vi "Settings cluster Broadcast.vi"(8 "error in (no error)":errorcluster, 10 "Settings cluster":T1={"Defaults"={"Default User"=0.0, "VISA Resource Name "="Tracker", "Histogram parameters"={"max"=300.0, "min"=0.0, "# bins"=10, "threshold"=8.0, "thr. type"=enum."higher accepted"}}, "Recording and saving"={"Researcher name"="Researcher", "Name prefix"="Track", "Data post-processing"={"Filter type"=enum."Savitzky-Golay", "Length"=31, "Order"=3}, "Stop at"=0.0, "\"Stop at\" enabled"=FALSE, "Default save folder path"=path "", "Acquisition FPS"=enum."Max"}, "Geometry"={"Sensor board size"=enum."Large", "Bridge swap"=FALSE, "Twisted neck"=FALSE, "Bridge H. offset"=30.0, "Bridge V. offset"=75.0, "Magnets orientation"=0.0, "Cage type"=0, "Cage parameters"={"Round"=variant, "Square"=variant, "Donut-maze"=variant, "T-maze"=variant, "Sociability-maze"=variant}}, "IO parameters"={"IO general config."=12, "IO 1 configuration"=1, "IO 2 configuration"=1, "IO 3 configuration"=0, "IO 4 configuration"=0, "Activate ext. RS-232"=0, "IO inversion config."=0, "Sync capability"=1}, "Conditions presets array"=[{"Enabled"=FALSE, "Name"="", "Specifier(s)"=[], "Response"={"Response type"=enum."Air puff", "TTL port"=enum."Port 1", "TTL pulse length, ms"=0.0}, "Has been set"=FALSE}, {"Enabled"=FALSE, "Name"="", "Specifier(s)"=[], "Response"={"Response type"=enum."Air puff", "TTL port"=enum."Port 1", "TTL pulse length, ms"=0.0}, "Has been set"=FALSE}, {"Enabled"=FALSE, "Name"="", "Specifier(s)"=[], "Response"={"Response type"=enum."Air puff", "TTL port"=enum."Port 1", "TTL pulse length, ms"=0.0}, "Has been set"=FALSE}, {"Enabled"=FALSE, "Name"="", "Specifier(s)"=[], "Response"={"Response type"=enum."Air puff", "TTL port"=enum."Port 1", "TTL pulse length, ms"=0.0}, "Has been set"=FALSE}, {"Enabled"=FALSE, "Name"="", "Specifier(s)"=[], "Response"={"Response type"=enum."Air puff", "TTL port"=enum."Port 1", "TTL pulse length, ms"=0.0}, "Has been set"=FALSE}, {"Enabled"=FALSE, "Name"="", "Specifier(s)"=[], "Response"={"Response type"=enum."Air puff", "TTL port"=enum."Port 1", "TTL pulse length, ms"=0.0}, "Has been set"=FALSE}, {"Enabled"=FALSE, "Name"="", "Specifier(s)"=[], "Response"={"Response type"=enum."Air puff", "TTL port"=enum."Port 1", "TTL pulse length, ms"=0.0}, "Has been set"=FALSE}, {"Enabled"=FALSE, "Name"="", "Specifier(s)"=[], "Response"={"Response type"=enum."Air puff", "TTL port"=enum."Port 1", "TTL pulse length, ms"=0.0}, "Has been set"=FALSE}, {"Enabled"=FALSE, "Name"="", "Specifier(s)"=[], "Response"={"Response type"=enum."Air puff", "TTL port"=enum."Port 1", "TTL pulse length, ms"=0.0}, "Has been set"=FALSE}, {"Enabled"=FALSE, "Name"="", "Specifier(s)"=[], "Response"={"Response type"=enum."Air puff", "TTL port"=enum."Port 1", "TTL pulse length, ms"=0.0}, "Has been set"=FALSE}, {"Enabled"=FALSE, "Name"="", "Specifier(s)"=[], "Response"={"Response type"=enum."Air puff", "TTL port"=enum."Port 1", "TTL pulse length, ms"=0.0}, "Has been set"=FALSE}, {"Enabled"=FALSE, "Name"="", "Specifier(s)"=[], "Response"={"Response type"=enum."Air puff", "TTL port"=enum."Port 1", "TTL pulse length, ms"=0.0}, "Has been set"=FALSE}, {"Enabled"=FALSE, "Name"="", "Specifier(s)"=[], "Response"={"Response type"=enum."Air puff", "TTL port"=enum."Port 1", "TTL pulse length, ms"=0.0}, "Has been set"=FALSE}, {"Enabled"=FALSE, "Name"="", "Specifier(s)"=[], "Response"={"Response type"=enum."Air puff", "TTL port"=enum."Port 1", "TTL pulse length, ms"=0.0}, "Has been set"=FALSE}], "Calibration parameters"={"Timing calibration sw/hw"=1.0, "True FPS"=80.0, "True frame time, s"=0.0125, "Disp. calibration info"=[]}} {"Calibration parameters"."True frame time, s" format="%.10g"; "Calibration parameters"."Disp. calibration info"."Speed, µl per ms" format="%.3g"; "Calibration parameters"."True FPS" format="%.10g"; "Calibration parameters"."Timing calibration sw/hw" format="%.10g"; "Conditions presets array"."Specifier(s)"."Validity criteria(s)"."Validity value" min=0.0 step=0.1 format="%.2g"; "Conditions presets array"."Specifier(s)"."Value" step=1.0 format="%#.2g"; "Recording and saving"."Data post-processing"."Order" min=3 max=11 step=2; "Recording and saving"."Data post-processing"."Length" min=5 max=301 step=2; "Geometry"."Cage type" items=["Round", "Square", "Donut-maze", "T-maze", "Sociability maze", ""]}) -> (0 "error out":errorcluster)   [LabVIEW 2018, in "Settings.lvlib"]
doc: "Broadcasts event cluster to every subscribed module.\n_____\nCreated using Delacor QMH Event Scripter 4.2.1.88."
uses:
  Settings.lvlib
  Common/Typedefs/CTL_Settings_cluster_2.ctl
  SubVi's/Controls/CTL_Histogram_parameters.ctl
  SubVi's/Controls/CTL_Filter_selector.ctl
  SubVi's/Controls/CTL_Acquisition_speed_selector.ctl
  Common/Typedefs/CTL_Segmented_plot_parameters_2.ctl
  Cage Diagram/Typedefs/CTL_Cage_type.ctl
  SubVi's/Controls/CTL_Cage_all_segmentation_params_set.ctl
  SubVi's/Controls/CTL_IO_params_cluster.ctl
  SubVi's/Controls/CTL_Conditions_Array.ctl
  SubVi's/Controls/CTL_Conditions_Cluster.ctl
  SubVi's/Controls/CTL_Condition_type.ctl
  SubVi's/Controls/CTL_Comparison_type.ctl
  SubVi's/Controls/CTL_Validity_check_criteria.ctl
  SubVi's/Controls/CTL_Response_info.ctl
  SubVi's/Controls/CTL_Condition_response_type.ctl
  SubVi's/Controls/CTL_Reponse_port_info.ctl
  SubVi's/Controls/CTL_Calibration_parameters.ctl
  SubVi's/Controls/CTL_Dispenser_calibration_info.ctl
  Settings cluster Broadcast Argument--cluster.ctl
  Common_Resources.lvlib
  Cage Diagram/Cage Diagram.lvlib
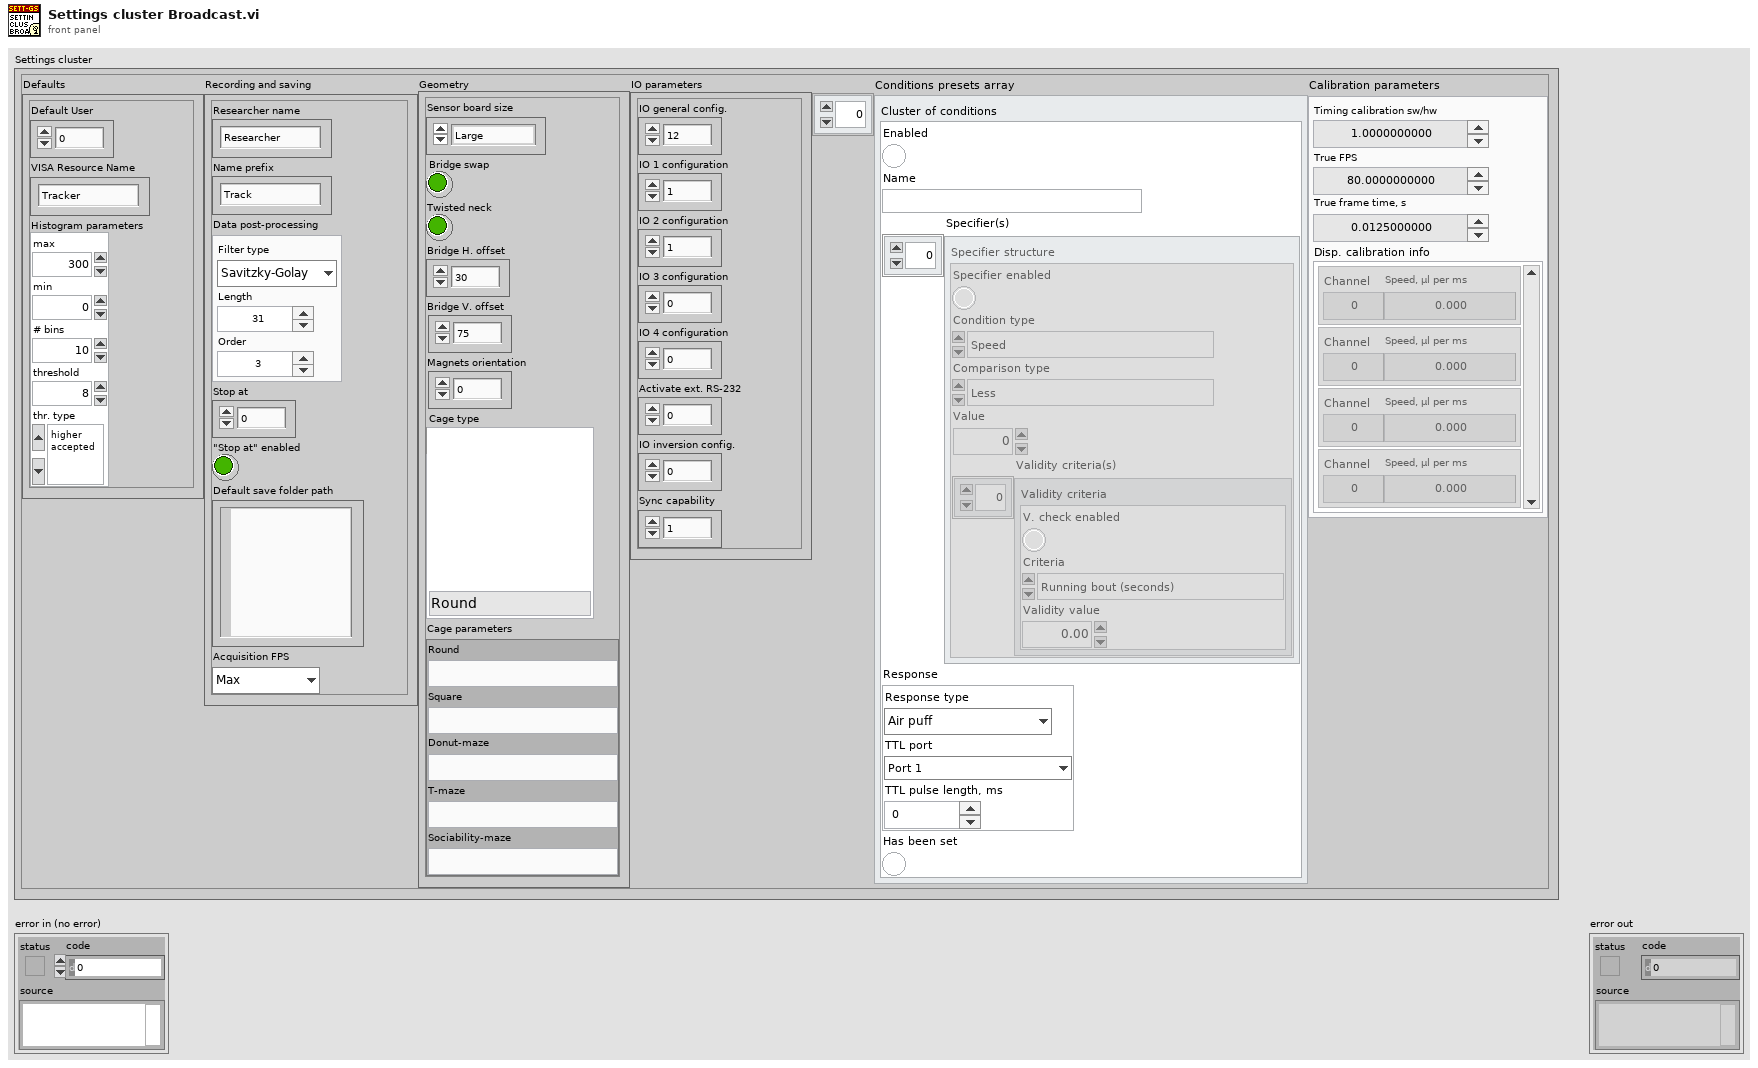
[diagram p1: front panel]
types:
  T1 = typedef "Common_Resources.lvlib/CTL_Settings_cluster_2.ctl" = cluster{"Defaults":cluster{"Default User":dbl, "VISA Resource Name ":string, "Histogram parameters":T2}, "Recording and saving":cluster{"Researcher name":string, "Name prefix":string, "Data post-processing":T3, "Stop at":dbl, "\"Stop at\" enabled":bool, "Default save folder path":path, "Acquisition FPS":T4}, "Geometry":T5, "IO parameters":T8, "Conditions presets array":T9, "Calibration parameters":T17}
  T2 = typedef "Common_Resources.lvlib/CTL_Histogram_parameters.ctl" = cluster{"max":dbl, "min":dbl, "# bins":i32, "threshold":dbl, "thr. type":enum16{"higher accepted", "lower accepted"}}
  T3 = typedef "Common_Resources.lvlib/CTL_Filter_selector.ctl" = cluster{"Filter type":enum16{"None", "Savitzky-Golay"}, "Length":i32, "Order":i32}
  T4 = typedef "Common_Resources.lvlib/CTL_Acquisition_speed_selector.ctl" = enum16{"Max", "Optimal", "Eco"}
  T5 = typedef "Common_Resources.lvlib/CTL_Segmented_plot_parameters_2.ctl" = cluster{"Sensor board size":enum16{"", "Large"}, "Bridge swap":bool, "Twisted neck":bool, "Bridge H. offset":sgl, "Bridge V. offset":sgl, "Magnets orientation":sgl, "Cage type":T6, "Cage parameters":T7}
  T6 = typedef "Cage Diagram.lvlib/CTL_Cage_type.ctl" = u16
  T7 = typedef "Common_Resources.lvlib/CTL_Cage_all_segmentation_params_set.ctl" = cluster{"Round":variant, "Square":variant, "Donut-maze":variant, "T-maze":variant, "Sociability-maze":variant}
  T8 = typedef "Common_Resources.lvlib/CTL_IO_params_cluster.ctl" = cluster{"IO general config.":u16, "IO 1 configuration":u16, "IO 2 configuration":u16, "IO 3 configuration":u16, "IO 4 configuration":u16, "Activate ext. RS-232":u16, "IO inversion config.":u16, "Sync capability":u8}
  T9 = typedef "Common_Resources.lvlib/CTL_Conditions_Array.ctl" = T10[]
  T10 = typedef "Common_Resources.lvlib/CTL_Conditions_Cluster.ctl" = cluster{"Enabled":bool, "Name":string, "Specifier(s)":cluster{"Specifier enabled":bool, "Condition type":T11, "Comparison type":T12, "Value":dbl, "Validity criteria(s)":cluster{"V. check enabled":bool, "Criteria":T13, "Validity value":dbl}[]}[], "Response":T14, "Has been set":bool}
  T11 = typedef "Common_Resources.lvlib/CTL_Condition_type.ctl" = enum16{"Speed", "Zone", "Angle to wall"}
  T12 = typedef "Common_Resources.lvlib/CTL_Comparison_type.ctl" = enum16{"Less", "Less or Equal", "Equal", "Greater or Equal", "Greater", "Not Equal"}
  T13 = typedef "Common_Resources.lvlib/CTL_Validity_check_criteria.ctl" = enum16{"Running bout (seconds)", "Running bout (meters)"}
  T14 = typedef "Common_Resources.lvlib/CTL_Response_info.ctl" = cluster{"Response type":T15, "TTL port":T16, "TTL pulse length, ms":dbl}
  T15 = typedef "Common_Resources.lvlib/CTL_Condition_response_type.ctl" = enum16{"None", "Air puff", "Liquid reward", "TTL pulse", "TTL pulse (ubr)", "TTL signal"}
  T16 = typedef "Common_Resources.lvlib/CTL_Reponse_port_info.ctl" = enum16{"Port 1", "Port 2", "Port 3", "Port 4"}
  T17 = typedef "Common_Resources.lvlib/CTL_Calibration_parameters.ctl" = cluster{"Timing calibration sw/hw":dbl, "True FPS":dbl, "True frame time, s":dbl, "Disp. calibration info":T18}
  T18 = typedef "Common_Resources.lvlib/CTL_Dispenser_calibration_info.ctl" = cluster{"Channel":u8, "Speed, µl per ms":dbl}[]
  T19 = typedef "Settings.lvlib/Settings cluster Broadcast Argument--cluster.ctl" = cluster{"Settings cluster":T1}
  T20 = typedef "Settings.lvlib/Broadcast Events--cluster.ctl" = cluster{"Module Did Init":refnum<user-event>, "Status Updated":refnum<user-event>, "Error Reported":refnum<user-event>, "Module Did Stop":refnum<user-event>, "Update Module Execution Status":refnum<user-event>, "Settings cluster Broadcast":refnum<user-event>}
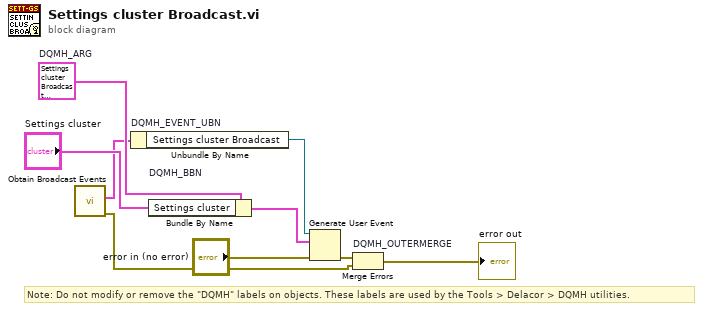
[diagram p0: block diagram]
diagram:
  w4 = T19 {"Settings cluster"={"Defaults"={"Default User"=0.0, "VISA Resource Name "="Tracker", "Histogram parameters"={"max"=300.0, "min"=0.0, "# bins"=10, "threshold"=8.0, "thr. type"=enum."higher accepted"}}, "Recording and saving"={"Researcher name"="Researcher", "Name prefix"="Track", "Data post-processing"={"Filter type"=enum."Savitzky-Golay", "Length"=31, "Order"=3}, "Stop at"=0.0, "\"Stop at\" enabled"=FALSE, "Default save folder path"=path "", "Acquisition FPS"=enum."Max"}, "Geometry"={"Sensor board size"=enum."Large", "Bridge swap"=FALSE, "Twisted neck"=FALSE, "Bridge H. offset"=30.0, "Bridge V. offset"=75.0, "Magnets orientation"=0.0, "Cage type"=0, "Cage parameters"={"Round"=variant, "Square"=variant, "Donut-maze"=variant, "T-maze"=variant, "Sociability-maze"=variant}}, "IO parameters"={"IO general config."=12, "IO 1 configuration"=1, "IO 2 configuration"=1, "IO 3 configuration"=0, "IO 4 configuration"=0, "Activate ext. RS-232"=0, "IO inversion config."=0, "Sync capability"=1}, "Conditions presets array"=[{"Enabled"=FALSE, "Name"="", "Specifier(s)"=[], "Response"={"Response type"=enum."Air puff", "TTL port"=enum."Port 1", "TTL pulse length, ms"=0.0}, "Has been set"=FALSE}, {"Enabled"=FALSE, "Name"="", "Specifier(s)"=[], "Response"={"Response type"=enum."Air puff", "TTL port"=enum."Port 1", "TTL pulse length, ms"=0.0}, "Has been set"=FALSE}, {"Enabled"=FALSE, "Name"="", "Specifier(s)"=[], "Response"={"Response type"=enum."Air puff", "TTL port"=enum."Port 1", "TTL pulse length, ms"=0.0}, "Has been set"=FALSE}, {"Enabled"=FALSE, "Name"="", "Specifier(s)"=[], "Response"={"Response type"=enum."Air puff", "TTL port"=enum."Port 1", "TTL pulse length, ms"=0.0}, "Has been set"=FALSE}, {"Enabled"=FALSE, "Name"="", "Specifier(s)"=[], "Response"={"Response type"=enum."Air puff", "TTL port"=enum."Port 1", "TTL pulse length, ms"=0.0}, "Has been set"=FALSE}, {"Enabled"=FALSE, "Name"="", "Specifier(s)"=[], "Response"={"Response type"=enum."Air puff", "TTL port"=enum."Port 1", "TTL pulse length, ms"=0.0}, "Has been set"=FALSE}, {"Enabled"=FALSE, "Name"="", "Specifier(s)"=[], "Response"={"Response type"=enum."Air puff", "TTL port"=enum."Port 1", "TTL pulse length, ms"=0.0}, "Has been set"=FALSE}, {"Enabled"=FALSE, "Name"="", "Specifier(s)"=[], "Response"={"Response type"=enum."Air puff", "TTL port"=enum."Port 1", "TTL pulse length, ms"=0.0}, "Has been set"=FALSE}, {"Enabled"=FALSE, "Name"="", "Specifier(s)"=[], "Response"={"Response type"=enum."Air puff", "TTL port"=enum."Port 1", "TTL pulse length, ms"=0.0}, "Has been set"=FALSE}, {"Enabled"=FALSE, "Name"="", "Specifier(s)"=[], "Response"={"Response type"=enum."Air puff", "TTL port"=enum."Port 1", "TTL pulse length, ms"=0.0}, "Has been set"=FALSE}, {"Enabled"=FALSE, "Name"="", "Specifier(s)"=[], "Response"={"Response type"=enum."Air puff", "TTL port"=enum."Port 1", "TTL pulse length, ms"=0.0}, "Has been set"=FALSE}, {"Enabled"=FALSE, "Name"="", "Specifier(s)"=[], "Response"={"Response type"=enum."Air puff", "TTL port"=enum."Port 1", "TTL pulse length, ms"=0.0}, "Has been set"=FALSE}, {"Enabled"=FALSE, "Name"="", "Specifier(s)"=[], "Response"={"Response type"=enum."Air puff", "TTL port"=enum."Port 1", "TTL pulse length, ms"=0.0}, "Has been set"=FALSE}, {"Enabled"=FALSE, "Name"="", "Specifier(s)"=[], "Response"={"Response type"=enum."Air puff", "TTL port"=enum."Port 1", "TTL pulse length, ms"=0.0}, "Has been set"=FALSE}], "Calibration parameters"={"Timing calibration sw/hw"=1.0, "True FPS"=80.0, "True frame time, s"=0.0125, "Disp. calibration info"=[]}}}  # DQMH_ARG
  # "Note: Do not modify or remove the \"DQMH\" labels on objects. These labels are used by the Tools > Delacor > DQMH utilities."
  n1 = call "Obtain Broadcast Events.vi"() -> ("error out"=w2:errorcluster, "Settings Broadcast Events"=w1:T20)  [unwired: 10 in]
  n2 = Unbundle By Name "DQMH_EVENT_UBN"(w1) -> ("Settings cluster Broadcast"=w6:refnum<user-event>)
  n3 = Bundle By Name "DQMH_BBN"(cluster=w4, "Settings cluster"="Settings cluster") -> (w7:T19)
  n4 = Generate User Event(user event=w6, event data cluster=w7, error in="error in (no error)") -> (error out=w5:errorcluster)  [unwired: 1 in, 1 out]
  n5 = Merge Errors "DQMH_OUTERMERGE"(w5, w2) -> (→"error out":errorcluster)
